vi "Example.vi"() -> ()   [LabVIEW 2015]
uses:
  lvlib/LV_CloudTranslationAPI.lvlib
panel:
  in  "To":string(combo)="ja"
  in  "accesskey":string
  out "翻訳結果":string[](array[string])
  in  "テキスト":string
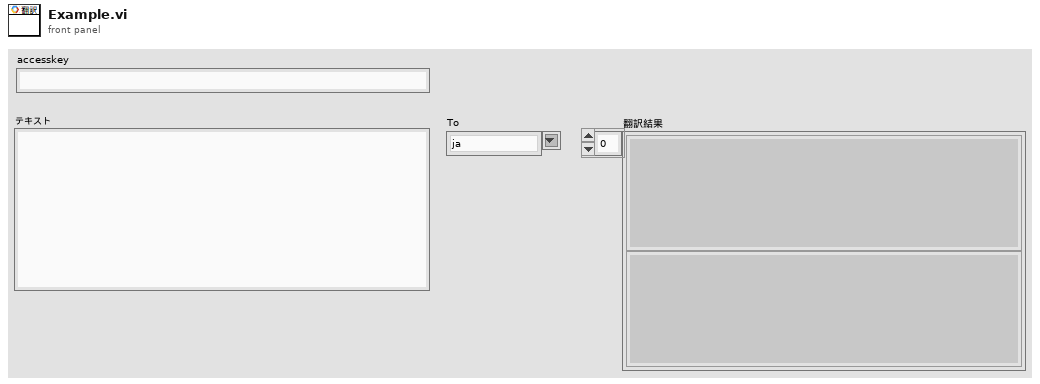
[diagram p1: front panel]
types:
  T1 = typedef "LV_CloudTranslationAPI.lvlib/Handler.ctl" = cluster{"http client handle":T2, "Base URL":string, "HMACSHA256":refnum<k24>, "API key":string, "Token Expiration ":timestamp}
  T2 = typedef "LabVIEWHTTPClient.lvlib/ClientHandle.ctl" = refnum<k1>
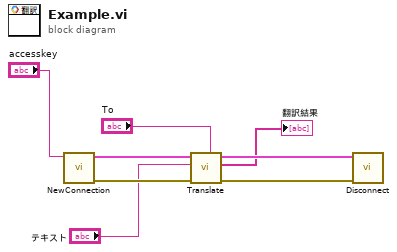
[diagram p0: block diagram]
diagram:
  n1 = call "NewConnection.vi"("accesskey"="accesskey") -> ("error out"=w6:errorcluster, "Handler out"=w7:T1)  [unwired: 9 in]
  n2 = call "Translate.vi"("To"="To", "error in"=w6, "テキスト"="テキスト", "Handler"=w7) -> ("error out"=w3:errorcluster, "翻訳結果"=→"翻訳結果":string[], "Handler out"=w4:T1)  [unwired: 4 in, 1 out]
  n3 = call "Disconnect.vi"("エラー入力（エラーなし）"=w3, "Handler out"=w4) -> ()  [unwired: 9 in, 1 out]
